vi "SwissSPAD Live_Save SS2 Data to HDF5_DVI.vi"(4 "Compression Level (0-9)":u8=9 max=9, 6 "Compression":bool, 7 "10-bit Gate Image":bool, 8 "error in (no error)":errorcluster, 9 "File Path::n":string="SS2 Live Gate Data Q", 11 "HDF5 ref":T1 format="%.0x") -> (0 "error out":errorcluster)   [LabVIEW 2021]
uses:
  <vilib>/addons/h5labview2/base/hid_t.ctl
  SwissSPAD Live_SS2 DAQ Parameters 3.ctl
  SwissSPAD Live_SS2 Gate Definition.ctl
  SwissSPAD Live_Settings List.ctl
  <vilib>/addons/h5labview2/file/H5F.lvlib
  <vilib>/addons/h5labview2/group/H5G.lvlib
  Notebook/Notebook.lvlib
  Rich Text Box/Rich Text Box.lvlib
  Variant/Variant to Data/Variant to Data.lvlib
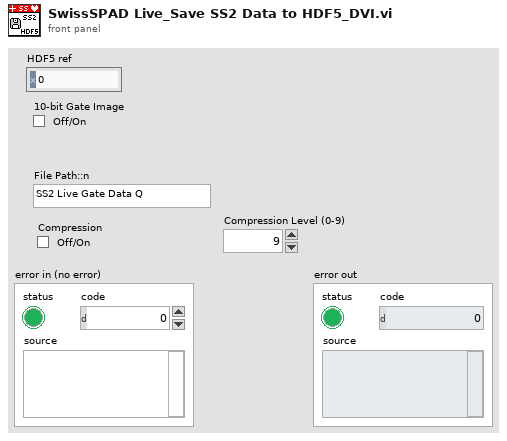
[diagram p1: front panel]
types:
  T1 = typedef "hid_t.ctl" = i32
  T2 = typedef "SwissSPAD Live_SS2 DAQ Parameters 3.ctl" = cluster{"10 bits":bool, "# Exposure Sequences":u32, "# 1-bit Frame per Gate":u32, "Gate Shift":u32, "# Gates per Set":u32, "# Sets":u32, "Laser Period":dbl[unit], "Sync Period":dbl[unit], "Gate Offset":u32, "Auto-adjust Gate Offset":bool, "Gate Definition":T3, "Reversed Shift":bool}
  T3 = typedef "SwissSPAD Live_SS2 Gate Definition.ctl" = cluster{"gs_psincdec_0":u32, "gs_psincdec_1":u32, "gs_psincdec_2":u32, "gs_psincdec_3":u32, "gs_no_shift_adj_1":u32, "gs_no_shift_adj_2":u32, "gs_no_shift_adj_3":u32}
  T4 = typedef "SwissSPAD Live_Settings List.ctl" = enum16{"FPGA:Bottom Half", "FPGA:Top Half", "FPGA:Bottom Bitfile Path", "FPGA:Top Bitfile Path", "FPGA:Bottom Bitstream Version", "FPGA:Top Bitstream Version", "FPGA:Auto Reset FPGA", "FPGA:Bottom FPGA Serial Number", "FPGA:Top FPGA Serial Number", "FPGA:Detector PCB Version", "Acquisition Parameters:Microlens", "Acquisition Parameters:SS2 DAQ Parameters", "Acquisition Parameters:Gate Configuration Array", "Acquisition Parameters:SS3 DAQ Parameters", "Acquisition Parameters:Buffer Size (# 8-bit Gates)", "File Information:File Information", "File Information:# Datasets in Series", "File Information:Scrambled File Flag", "File Information:SS3 Gate Slip Correction", "File Information:SS3 Hot Pixel Mismatch Detection", "File Information:Delay between Datasets", "File Information:Save Sum of All Gates Preview", "Image Parameters:Image ROI Information", "Image Parameters:Image Binning Options", "Image Parameters:SS3 Displayed Image", "Image Parameters:Image Display Options", "Image Parameters:Use Histogram Cursors", "Image Parameter:FPGA Data to Display", "UI Settings:Histogram Bins Number", "UI Settings:Use Image Display Options", "UI Settings:Verbose Settings", "UI Settings:Verbose Saving"}
  T5 = typedef "SwissSPAD Live_File Saving Task Information.ctl" = cluster{"File Path::n":string, "# Saved Images":i32, "# Images (Total)":i32, "File Size (Bytes)":i64}
  T6 = typedef "Rich Text Box.lvlib/Text Formatting.ctl" = cluster{"Font":string, "Text Color":T7, "Text Background Color":T7, "Text Style":enum16{"Regular", "Bold", "Italic", "Underline", "Strikeout"}, "Font Size (Points)":dbl, "Text Alignment":i32}
  T7 = typedef "Rich Text Box.lvlib/Text Colors.ctl" = enum16{"Unchanged", "Black", "Blue", "Brown", "Gray", "Green", "Orange", "Pink", "Red", "White"}
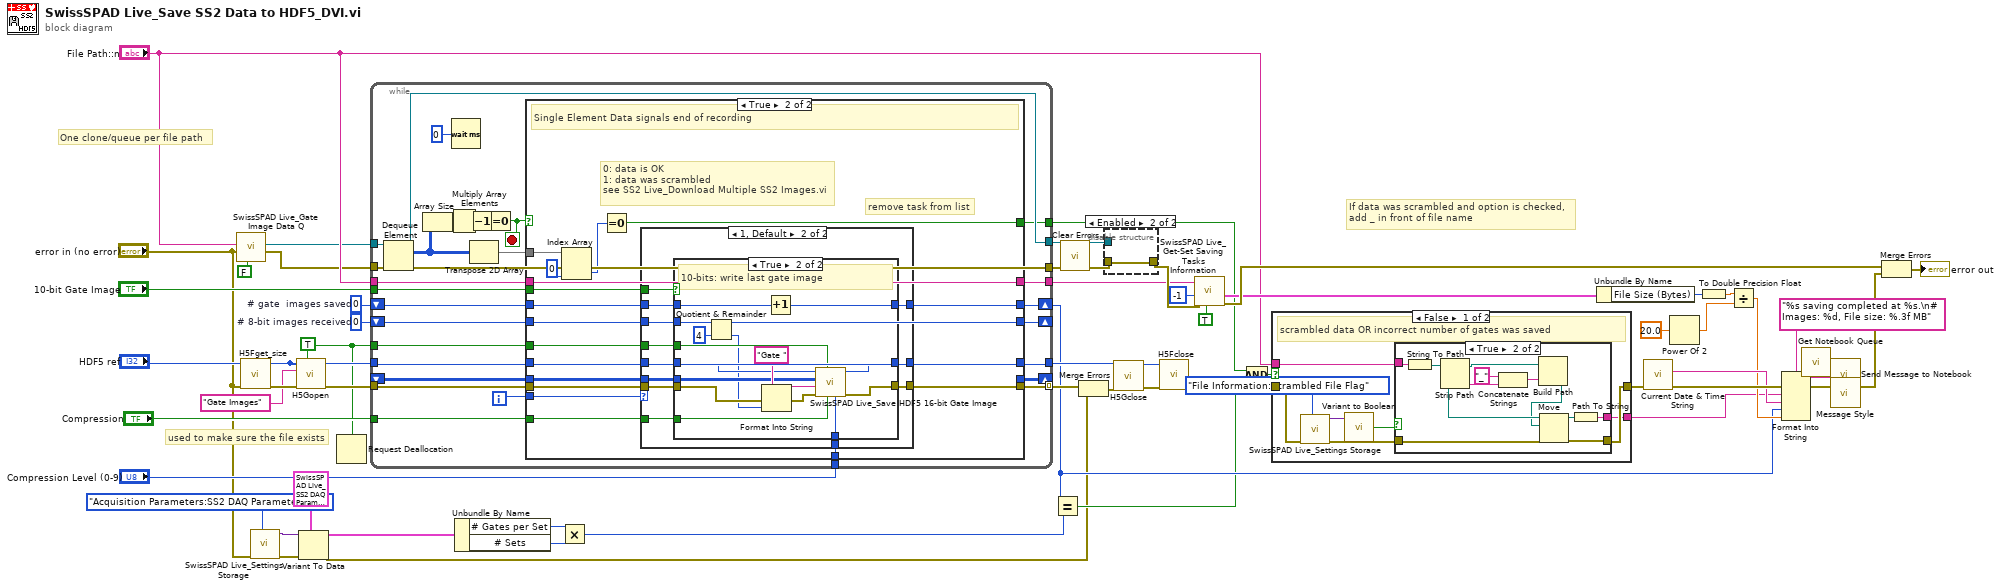
[diagram p0: block diagram]
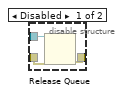
[diagram p2: hidden frame]
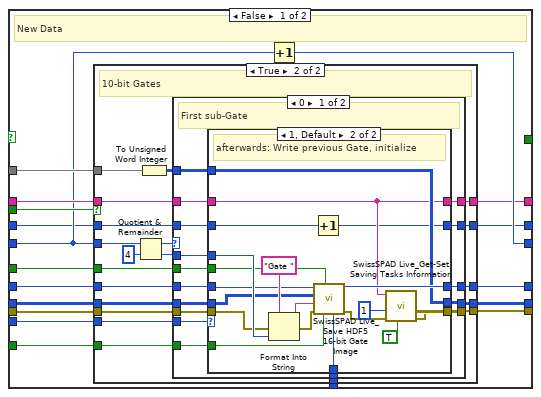
[diagram p5: hidden frame]
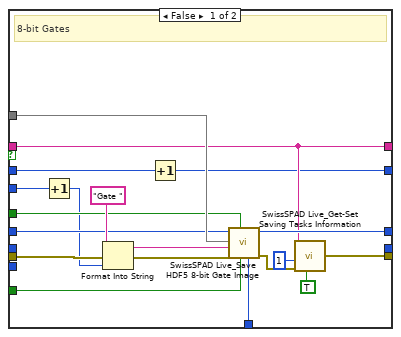
[diagram p6: hidden frame]
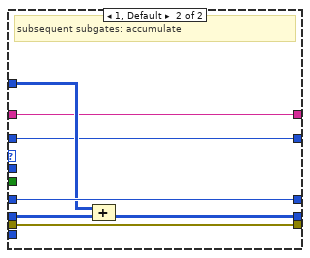
[diagram p8: hidden frame]
diagram:
  w18 = 0  # # gate  images saved
  w31 = TRUE ("create? (F)")
  w59 = 0  # # 8-bit images received
  # "If data was scrambled and option is checked,\nadd _ in front of file name"
  # "One clone/queue per file path"
  # "used to make sure the file exists"
  n1 = call "SwissSPAD Live_Gate Image Data Q.vi"("create if not found? (T)"=FALSE, "error in (no error)"="error in (no error)", "SwissSPAD Live Gate Image Data Q Name"="File Path::n") -> ("error out"=w4:errorcluster, "SwissSPAD Live Gate Image Data Q"=w6:refnum<queue>)  [unwired: 6 in, 1 out]
  n2 = call <vilib>:"H5Fget_size.vi"("error in (no error)"="error in (no error)", "ref in"="HDF5 ref") -> ("error out"=w58:errorcluster, "ref out"=w51:T1)  [unwired: 7 in, 1 out]
  n3 = call "SwissSPAD Live_Settings Storage.vi"("Settings List"=SwissSPAD_Live_Settings_List."Acquisition Parameters:SS2 DAQ Parameters", "Error In"="error in (no error)") -> ("Error Out"=w17:errorcluster, "Variant Data out"=w1:variant)  [unwired: 8 in]
  n4 = call <vilib>:"H5Gopen.vi"("create? (F)"=w31, "error in (no error)"=w58, "name"="Gate Images", "ref in"=w51) -> ("error out"=w57:errorcluster, "group out"=w55:T1)  [unwired: 6 in]
  n5 = Variant To Data(error in=w17, type=T2 {"10 bits"=FALSE, "# Exposure Sequences"=0, "# 1-bit Frame per Gate"=0, "Gate Shift"=0, "# Gates per Set"=0, "# Sets"=1, "Laser Period"=0.0, "Sync Period"=0.0, "Gate Offset"=0, "Auto-adjust Gate Offset"=FALSE, "Gate Definition"={"gs_psincdec_0"=0, "gs_psincdec_1"=0, "gs_psincdec_2"=0, "gs_psincdec_3"=0, "gs_no_shift_adj_1"=0, "gs_no_shift_adj_2"=0, "gs_no_shift_adj_3"=0}, "Reversed Shift"=FALSE} ("SS2 DAQ Parameters"), Variant=w1) -> (data=w16:T2, error out=w8:errorcluster)
  n6 = Request Deallocation(w31) -> ()
  n7 = while {
    tunnel: w6 -> [w89]
    tunnel: [w88] -> w60
    tunnel: w55 -> [w87]
    tunnel: w57 -> [w71]
    shift-right: [w79] -> _
    shift-left: w59 -> [w86]
    tunnel: w31 -> [w85]
    tunnel: [w84] -> w54 mode=indexing
    tunnel: [w83] -> w53
    tunnel: "10-bit Gate Image" -> [w77]
    shift-right: [w75] -> _
    shift-left: _ -> [w76]
    tunnel: [w73] -> w49
    tunnel: w4 -> [w70]
    tunnel: "File Path::n" -> [w69]
    tunnel: "Compression" -> [w68]
    tunnel: [w67] -> w25
    tunnel: [w65] -> w23
    tunnel: "Compression Level (0-9)" -> [w64]
    shift-right: [w62] -> w12
    shift-left: w18 -> [w63]
    i -> [w74]
    stop <- w80 stop-if-true
    n8 = Dequeue Element(queue=w89, error in (no error)=w70) -> (queue out=w88:refnum<queue>, element=w78:u8[][], error out=w73:errorcluster)  [unwired: 1 in, 1 out]
    n9 = Array Size(array=w78) -> (size(s)=w81:i32[])
    n10 = Multiply Array Elements(1:w81) -> (0:w82:i32)
    n11 = Wait (ms)(milliseconds to wait=u32 0) -> ()  [unwired: 1 out]
    n12 = Decrement(x=w82) -> (x-1=w66:i32)
    n13 = Transpose 2D Array(2D array=w78) -> (transposed array=w72:u8[][])
    n14 = Equal To 0?(x=w66) -> (x = 0?=w80:bool)
    n15 = case shown="True" w80 {
      tunnel: w87 -> [w106 w210]
      tunnel: w71 -> [w103 w208]
      tunnel: w86 -> [w95 w207]
      tunnel: w85 -> [w107 w205]
      tunnel: [w97 w202] -> w84
      tunnel: [w105 w209] -> w83
      tunnel: [w104 w207] -> w79
      tunnel: w72 -> [w101 w200]
      tunnel: w77 -> [w102 w206]
      tunnel: w76 -> [w100 w211]
      tunnel: [w99 _] -> w75
      tunnel: w74 -> [w98 w203]
      tunnel: w69 -> [w96 w201]
      tunnel: w68 -> [w94 w204]
      tunnel: [w93 w201] -> w67
      tunnel: [_ w197] -> w65
      tunnel: w64 -> [w92 w196]
      tunnel: w63 -> [w91 w195]
      tunnel: [w90 w194] -> w62
      frame False {
        # "New Data"
        n16 = case shown="True" w102 {
          tunnel: w107 -> [w118 w143]
          tunnel: [w115 w141] -> w97
          tunnel: w106 -> [w120 w145]
          tunnel: [w119 w144] -> w105
          tunnel: w103 -> [w126 w142]
          tunnel: w95 -> [w124 w132]
          tunnel: w101 -> [w121 w146]
          tunnel: w100 -> [_ w139]
          tunnel: [_ w137] -> w99
          tunnel: w98 -> [_ w140]
          tunnel: w96 -> [w111 w136]
          tunnel: w94 -> [w112 w131]
          tunnel: [w111 w130] -> w93
          tunnel: w92 -> [w110 w129]
          tunnel: w91 -> [w109 w128]
          tunnel: [w108 w127] -> w90
          frame False {
            # "8-bit Gates"
            n17 = Increment(x=w124) -> (x+1=w117:i32)
            n18 = Format Into String(initial string="Gate ", error in=w126, w117) -> (resulting string=w122:string, error out=w123:errorcluster)  [unwired: 1 in]
            n19 = Increment(x=w109) -> (x+1=w108:i32)
            n20 = call "SwissSPAD Live_Save HDF5 8-bit Gate Image.vi"("Compression Level (0-9)"=w110, "Compression"=w112, "Replace?"=w118, "error in (no error)"=w123, "Image Name"=w122, "Data"=w121, "ref in"=w120) -> ("error out"=w116:errorcluster, "ref out"=w119:T1)  [unwired: 3 in]
            n21 = call "SwissSPAD Live_Get-Set Saving Tasks Information.vi"("Get (F)/Set"=TRUE, "error in (no error)"=w116, "# New Images Saved (1)"=1 ("# New Images Saved"), "File Path::n"=w111) -> ("error out"=w115:errorcluster)  [unwired: 4 in, 3 out]
          }
          frame True {
            # "10-bit Gates"
            n22 = Quotient & Remainder(x=w132, y=4) -> (x-y*floor(x/y)=w133:i32, floor(x/y)=w134:i32)
            n23 = To Unsigned Word Integer(number=w146) -> (unsigned 16bit integer=w138:u16[][])
            n24 = case shown="0" w133 {
              tunnel: w145 -> [w162 w192]
              tunnel: [w161 w192] -> w144
              tunnel: w143 -> [w160 _]
              tunnel: w142 -> [w159 w193]
              tunnel: [w158 w193] -> w141
              tunnel: w140 -> [w157 _]
              tunnel: w134 -> [w156 _]
              tunnel: w139 -> [w154 w191]
              tunnel: w138 -> [w155 w190]
              tunnel: [w153 w189] -> w137
              tunnel: w136 -> [w152 w188]
              tunnel: w131 -> [w151 _]
              tunnel: [w150 w188] -> w130
              tunnel: w129 -> [w149 _]
              tunnel: w128 -> [w148 w187]
              tunnel: [w147 w187] -> w127
              frame 0 {
                # "First sub-Gate"
                n25 = case shown="1, Default" w157 {
                  tunnel: w162 -> [w167 w181]
                  tunnel: [w167 w186] -> w161
                  tunnel: w160 -> [_ w180]
                  tunnel: w159 -> [w166 w182]
                  tunnel: [w166 w175] -> w158
                  tunnel: w156 -> [_ w184]
                  tunnel: w155 -> [w165 w177]
                  tunnel: [w165 w177] -> w153
                  tunnel: w154 -> [_ w178]
                  tunnel: w152 -> [w164 w171]
                  tunnel: w151 -> [_ w172]
                  tunnel: [w164 w171] -> w150
                  tunnel: w149 -> [_ w170]
                  tunnel: w148 -> [w163 w169]
                  tunnel: [w163 w168] -> w147
                  frame 0 {
                    # "First Call: initialize"
                  }
                  frame 1, Default {
                    # "afterwards: Write previous Gate, initialize"
                    n26 = Format Into String(initial string="Gate ", error in=w182, w184) -> (resulting string=w179:string, error out=w183:errorcluster)  [unwired: 1 in]
                    n27 = Increment(x=w169) -> (x+1=w168:i32)
                    n28 = call "SwissSPAD Live_Save HDF5 16-bit Gate Image.vi"("Compression Level (0-9)"=w170, "Compression"=w172, "Replace?"=w180, "error in (no error)"=w183, "Image Name"=w179, "Data"=w178, "ref in"=w181) -> ("error out"=w176:errorcluster, "ref out"=w186:T1)  [unwired: 3 in]
                    n29 = call "SwissSPAD Live_Get-Set Saving Tasks Information.vi"("Get (F)/Set"=TRUE, "error in (no error)"=w176, "# New Images Saved (1)"=1, "File Path::n"=w171) -> ("error out"=w175:errorcluster)  [unwired: 4 in, 3 out]
                  }
                }
              }
              frame 1, Default {
                # "subsequent subgates: accumulate"
                n30 = Compound Arithmetic op=ADD(w190, w191) -> (w189:u16[][])
              }
            }
          }
        }
        n31 = Increment(x=w95) -> (x+1=w104:i32)
      }
      frame True {
        w199 = 0 ("index (row)")
        # "0: data is OK\n1: data was scrambled\nsee SS2 Live_Download Multiple SS2 Images.vi"
        # "remove task from list"
        # "Single Element Data signals end of recording"
        n32 = Index Array(array=w200, index (row)=w199, index (col)=w199) -> (element=w198:u8)
        n33 = Equal To 0?(x=w198) -> (x = 0?=w197:bool)
        n34 = case shown="1, Default" w203 {
          tunnel: w211 -> [_ w226]
          tunnel: w210 -> [w214 w225]
          tunnel: [w214 w224] -> w209
          tunnel: w208 -> [w213 w223]
          tunnel: w207 -> [_ w222]
          tunnel: [w213 w221] -> w202
          tunnel: w206 -> [_ w220]
          tunnel: w205 -> [_ w219]
          tunnel: w204 -> [_ w218]
          tunnel: w196 -> [_ w217]
          tunnel: w195 -> [w212 w216]
          tunnel: [w212 w215] -> w194
          frame 0 {
            # "no data ever received (FPGA timeout?)"
          }
          frame 1, Default {
            n35 = case shown="True" w220 {
              tunnel: w226 -> [_ w242]
              tunnel: w225 -> [w229 w241]
              tunnel: [w229 w240] -> w224
              tunnel: w223 -> [w228 w239]
              tunnel: [w228 w238] -> w221
              tunnel: w222 -> [_ w235]
              tunnel: w219 -> [_ w237]
              tunnel: w218 -> [_ w233]
              tunnel: w217 -> [_ w232]
              tunnel: w216 -> [w227 w231]
              tunnel: [w227 w230] -> w215
              frame False {
                # "8-bit data: nothing to do"
              }
              frame True {
                # "10-bits: write last gate image"
                n36 = Quotient & Remainder(x=w235, y=4) -> (floor(x/y)=w234:i32)  [unwired: 1 out]
                n37 = Format Into String(initial string="Gate ", error in=w239, w234) -> (resulting string=w243:string, error out=w244:errorcluster)  [unwired: 1 in]
                n38 = Increment(x=w231) -> (x+1=w230:i32)
                n39 = call "SwissSPAD Live_Save HDF5 16-bit Gate Image.vi"("Compression Level (0-9)"=w232, "Compression"=w233, "Replace?"=w237, "error in (no error)"=w244, "Image Name"=w243, "Data"=w242, "ref in"=w241) -> ("error out"=w238:errorcluster, "ref out"=w240:T1)  [unwired: 3 in]
              }
            }
          }
        }
      }
    }
  }
  n40 = Unbundle By Name(w16) -> ("# Gates per Set"=w14:u32, "# Sets"=w13:u32)
  n41 = Multiply(x=w14, y=w13) -> (x*y=w11:u32)
  n42 = Equal?(x=w12, y=w11) -> (x = y?=w9:bool)
  n43 = call <vilib>:"Clear Errors.vi"("error in (no error)"=w49) -> ("error out"=w24:errorcluster)  [unwired: 5 in, 1 out]
  n44 = Merge Errors(w54, w8) -> (w48:errorcluster)
  n45 = disable-structure shown="Enabled" {
    disable-tunnel: w60 -> [w248 _]
    disable-tunnel: [w247 w249] -> w28
    disable-tunnel: w24 -> [w246 w249]
    frame Disabled {
      n46 = Release Queue(queue=w248, error in (no error)=w246) -> (error out=w247:errorcluster)  [unwired: 1 in, 2 out]
    }
    frame Enabled {
    }
  }
  n47 = call <vilib>:"H5Gclose.vi"("error in (no error)"=w48, "group in"=w53) -> ("error out"=w52:errorcluster)  [unwired: 9 in]
  n48 = call <vilib>:"H5Fclose.vi"("error in (no error)"=w52, "ref"=w51) -> ("error out"=w22:errorcluster)  [unwired: 9 in]
  n49 = call "SwissSPAD Live_Get-Set Saving Tasks Information.vi"("Get (F)/Set"=TRUE, "error in (no error)"=w28, "# New Images Saved (1)"=-1 ("# New Images Saved"), "File Path::n"=w25) -> ("error out"=w27:errorcluster, "Complete Saving Task Information"=w26:T5)  [unwired: 4 in, 2 out]
  n50 = Compound Arithmetic op=AND(w23, w9) -> (w10:bool)
  n51 = case shown="False" w10 {
    tunnel: w22 -> [w257 w271]
    tunnel: [w253 w271] -> w21
    tunnel: "File Path::n" -> [w256 w272]
    tunnel: [w252 w272] -> w20
    frame False {
      # "scrambled data OR incorrect number of gates was saved"
      n52 = call "SwissSPAD Live_Settings Storage.vi"("Settings List"=SwissSPAD_Live_Settings_List."File Information:Scrambled File Flag", "Error In"=w257) -> ("Error Out"=w254:errorcluster, "Variant Data out"=w250:variant)  [unwired: 8 in]
      n53 = call "Variant to Boolean.vi"("Variant"=w250) -> ("Value"=w255:bool)  [unwired: 8 in]
      n54 = case shown="True" w255 {
        tunnel: w256 -> [w258 w270]
        tunnel: w254 -> [w259 w267]
        tunnel: [w259 w261] -> w253
        tunnel: [w258 w260] -> w252
        frame False {
        }
        frame True {
          n55 = String To Path(string=w270) -> (path=w266:path)
          n56 = Strip Path(path=w266) -> (stripped path=w265:path, name=w269:string)
          n57 = Concatenate Strings("_" ("string"), w269) -> (w264:string)
          n58 = Build Path(base path=w265, name or relative path=w264) -> (appended path=w263:path)
          n59 = Move(source path=w266, error in=w267, 10:w263) -> (error out=w261:errorcluster, 3:w262:path)  [unwired: 2 in, 1 out]
          n60 = Path To String(path=w262) -> (string=w260:string)
        }
      }
    }
    frame True {
      # "Data is not scrambled AND correct number of gates was saved"
    }
  }
  n61 = Unbundle By Name(w26) -> ("File Size (Bytes)"=w37:i64)
  n62 = call "Current Date & Time String.vi"("Error In"=w21) -> ("Error Out"=w39:errorcluster, "time string"=w38:string)  [unwired: 8 in, 1 out]
  n63 = Power Of 2(x=20.0) -> (2^x=w35:dbl)
  n64 = To Double Precision Float(number=w37) -> (double precision float=w33:dbl)
  n65 = Divide(x=w33, y=w35) -> (x/y=w34:dbl)
  n66 = Format Into String(format string="%s saving completed at %s.\n# Images: %d, File size: %.3f MB", error in=w39, w20, w38, w12, w34) -> (resulting string=w41:string, error out=w42:errorcluster)  [unwired: 1 in]
  n67 = call "Get Notebook Queue.vi"() -> ("Notebook Queue"=w45:refnum<queue>)  [unwired: 9 in]
  n68 = call "Message Style.vi"() -> ("Message Formatting"=w43:T6)
  n69 = call "Send Message to Notebook.vi"("Text Formatting"=w43, "Error In"=w42, "Message"=w41, "Notebook Queue"=w45) -> ("Error Out"=w44:errorcluster)  [unwired: 4 in, 1 out]
  n70 = Merge Errors(w27, w44) -> (→"error out":errorcluster)
